vi "Function Values.vi"(5 "result":dbl[][](array[numeric]) format="%.2f", 6 "list of variables":i32[](array[numeric])=[0, 0], 7 "table":i32[][][](array[numeric]), 9 "X":dbl[](array[numeric]) format="%.2f") -> (1 "F(X)":dbl[](array[numeric]) format="%.2f")   [LabVIEW 2020, in "NI_Gmath.lvlib"]
uses:
  NI_Gmath.lvlib
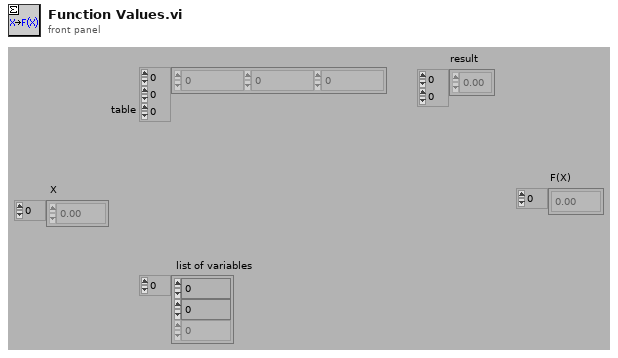
[diagram p1: front panel]
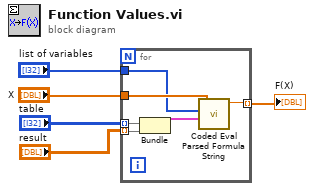
[diagram p0: block diagram]
diagram:
  n1 = for {
    tunnel: "X" -> [w10]
    tunnel: "result" -> [w7] mode=indexing
    tunnel: "table" -> [w8] mode=indexing
    tunnel: [w11] -> w4 mode=indexing
    tunnel: "list of variables" -> [w9]
    n2 = Bundle("table"=w8, "result"=w7) -> (w6:cluster{"table":i32[][], "result":dbl[]})  [unwired: 1 in]
    n3 = call "Coded Eval Parsed Formula String.vi"("Parsed Formula"=w6, "Variables"=w9, "X Values"=w10) -> ("y value"=w11:dbl)  [unwired: 1 in, 1 out]
  }
  "F(X)" <- w4
